vi "XML_Remove_Brackets.vi"(11 "Input String":string) -> (3 "String without brackets":string)   [LabVIEW 2011]
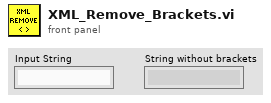
[diagram p1: front panel]
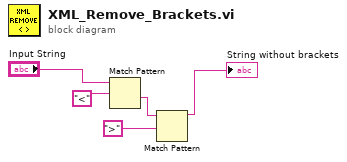
[diagram p0: block diagram]
diagram:
  n1 = Match Pattern(string="Input String", regular expression="<") -> (after substring=w3:string)  [unwired: 1 in, 3 out]
  n2 = Match Pattern(string=w3, regular expression=">") -> (before substring=→"String without brackets":string)  [unwired: 1 in, 3 out]
